vi "Funzioni array.vi"() -> ()   [LabVIEW 2012]
panel:
  out "1D array":dbl[](array[numeric])
  out "transposed array":dbl[][](array[numeric])
  out "decimated array 2":dbl[](array[numeric])
  out "decimated array":dbl[](array[numeric])
  out "interleaved array":dbl[](array[numeric])
  out "max index(es)":i32[](array[numeric])
  out "max value":dbl
  out "array con array sostituita":dbl[][](array[numeric])
  out "array con array inserita":dbl[][](array[numeric])
  out "array reshape":dbl[](array[numeric])
  out "sorted array":dbl[](array[numeric])
  out "split - second subarray":dbl[](array[numeric])
  out "split - first subarray":dbl[](array[numeric])
  out "index of element":i32
  out "subarray dalla riga (e prosegue per n righe)\ne dalla colonna (e prosegue per n colonne)":dbl[][](array[numeric])
  out "size(s)":i32[](array[numeric])
  out "deleted portion":dbl[][](array[numeric])
  out "array w/ subset deleted":dbl[][](array[numeric])
  out "reversed array":dbl[](array[numeric])
  out "subarray all'indice":dbl[](array[numeric])
  out "array (last n elements first)":dbl[](array[numeric])
  out "2D array":dbl[][](array[numeric])
  in  "N":i16=11
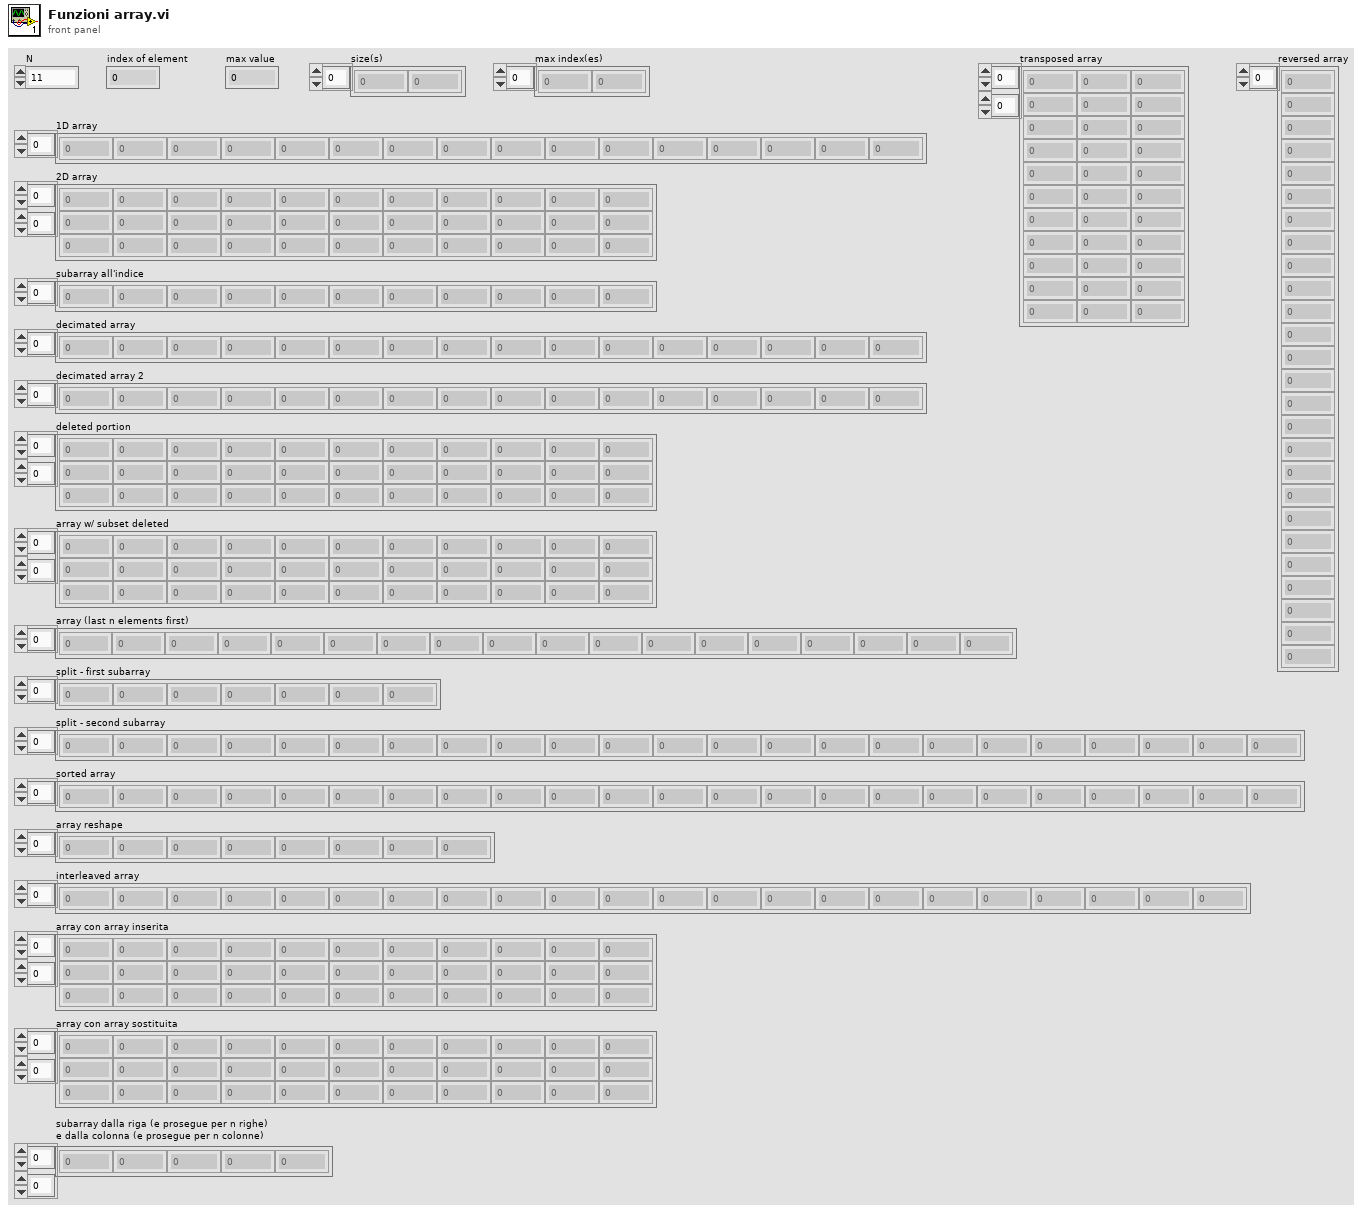
[diagram p1: front panel]
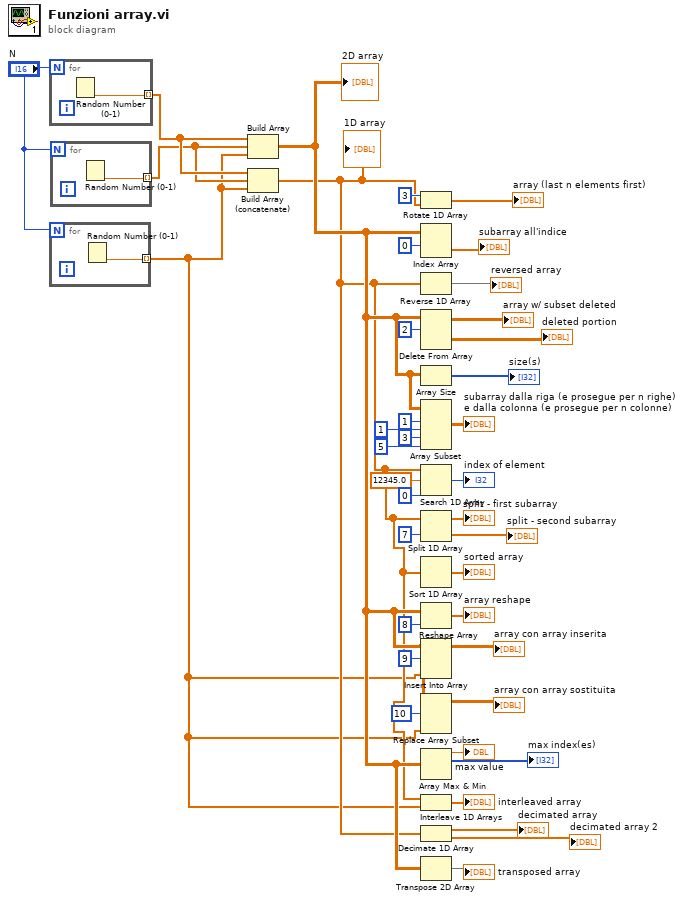
[diagram p0: block diagram]
diagram:
  n1 = for {
    N: "N" -> [_]
    tunnel: [w40] -> w38 mode=indexing
    n2 = Random Number (0-1)() -> (number: 0 to 1=w40:dbl)
  }
  n3 = for {
    N: "N" -> [_]
    tunnel: [w41] -> w6 mode=indexing
    n4 = Random Number (0-1)() -> (number: 0 to 1=w41:dbl)
  }
  n5 = for {
    N: "N" -> [_]
    tunnel: [w42] -> w37 mode=indexing
    n6 = Random Number (0-1)() -> (number: 0 to 1=w42:dbl)
  }
  n7 = Build Array(w38, w37, w6) -> (w36:dbl[][])
  "2D array" <- w36
  n8 = Build Array (concatenate)(w38, w37, w6) -> (w7:dbl[])
  "1D array" <- w7
  n9 = Rotate 1D Array(1:w7, 2:3 ("n")) -> (0:→"array (last n elements first)":dbl[])
  n10 = Index Array(array=w36, index (row)=0) -> (element=→"subarray all'indice":dbl[])  [unwired: 1 in]
  n11 = Reverse 1D Array(array=w7) -> (reversed array=→"reversed array":dbl[])
  n12 = Delete From Array(array=w36, length=2) -> (deleted portion=→"deleted portion":dbl[][], array with subset deleted=→"array w/ subset deleted":dbl[][])  [unwired: 2 in]
  n13 = Array Size(array=w36) -> (size(s)=→"size(s)":i32[])
  n14 = Array Subset(array=w36, index (row)=1 ("index"), length (row)=1 ("length"), index (col)=3 ("index"), length (col)=5 ("length")) -> (→"subarray dalla riga (e prosegue per n righe)\ne dalla colonna (e prosegue per n colonne)":dbl[][])
  n15 = Search 1D Array(1D array=w7, element=12345.0, start index (0)=0) -> (index of element=→"index of element":i32)
  n16 = Split 1D Array(array=w7, index=7) -> (first subarray=→"split - first subarray":dbl[], second subarray=→"split - second subarray":dbl[])
  n17 = Sort 1D Array(array=w7) -> (sorted array=→"sorted array":dbl[])
  n18 = Reshape Array(w36, 8 ("dimension size")) -> (→"array reshape":dbl[])
  n19 = Insert Into Array(array=w36, index (row)=9, new element=w6) -> (→"array con array inserita":dbl[][])  [unwired: 1 in]
  n20 = Replace Array Subset(array=w36, new element=w6, index (row)=10) -> (→"array con array sostituita":dbl[][])  [unwired: 1 in]
  n21 = Array Max & Min(array=w36) -> (max value=→"max value":dbl, max index (indices)=→"max index(es)":i32[])  [unwired: 2 out]
  n22 = Interleave 1D Arrays(w7, w6) -> (→"interleaved array":dbl[])
  n23 = Decimate 1D Array(w7) -> (→"decimated array":dbl[], →"decimated array 2":dbl[])
  n24 = Transpose 2D Array(2D array=w36) -> (transposed array=→"transposed array":dbl[][])
